vi "VG_TCellmin.vi"() -> ()   [LabVIEW 2020]
panel:
  out "TCellmin":dbl
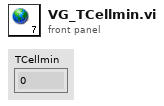
[diagram p1: front panel]
diagram:
